vi "Assign Value.vi"(8 "error in (no error)":errorcluster, 10 "Assigned Value":refnum<class "Abs_Value.lvclass">, 11 "Abs_Complex Double Float in":refnum<class "Abs_Complex Double Float.lvclass">) -> (0 "error out":errorcluster, 3 "Abs_Complex Double Float out":refnum<class "Abs_Complex Double Float.lvclass">)   [LabVIEW 2021, in "Abs_Complex Double Float.lvclass"]
uses:
  Abs_Complex Double Float.lvclass
  Value/Abs_Value.lvclass
  Numeric/Abs_Numeric.lvclass
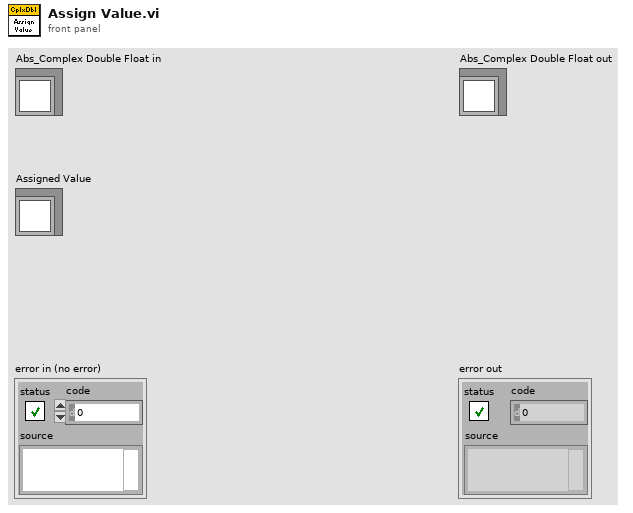
[diagram p1: front panel]
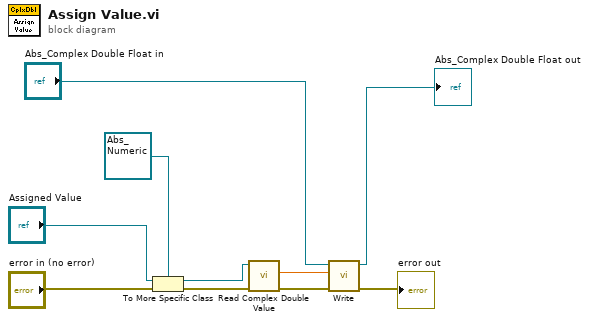
[diagram p0: block diagram]
diagram:
  n1 = To More Specific Class(target class=refnum<class "Abs_Numeric.lvclass"> refnum ("Abs_Numeric.lvclass"), reference="Assigned Value", error in="error in (no error)") -> (specific class reference=w6:refnum<class "Abs_Numeric.lvclass">, error out=w7:errorcluster)
  n2 = call-dynamic "Read Complex Double Value.vi"("error in (no error)"=w7, "Numeric in"=w6) -> ("error out"=w2:errorcluster, "Complex Double Float"=w1:cdb)  [unwired: 7 in, 1 out]
  n3 = call-dynamic "Write.vi"("error in (no error)"=w2, "Value"=w1, "Double Float.lvclass_340760 in"="Abs_Complex Double Float in") -> ("error out"=→"error out":errorcluster, "Double Float.lvclass_340760 out"=→"Abs_Complex Double Float out":refnum<class "Abs_Complex Double Float.lvclass">)  [unwired: 7 in]
